vi "Savitsky Golay Weighted Filter (multiple).vi"(4 "Window Order":i32, 6 "Side Points Unit (points)":enum16{"Points", "Data"}(ring), 8 "error in (no error)":errorcluster, 9 "polynomial order (3)":i32=3, 10 "side points (6)":dbl=6.0, 11 "XY-data":cluster{"X-array":dbl[], "Y-array":dbl[]}[](array[cluster])) -> (0 "error out":errorcluster, 3 "XY-data out":cluster{"X-array":dbl[], "Y-array":dbl[]}[](array[cluster]) {"Y-array" format="%.2p"; "X-array" format="%.2p"})   [LabVIEW 2019, in "xy_utilities.lvlib"]
doc: "Filter <b>XY-data</b>'s Y-Array with a Savitsky-Golay FIR smoothing filter.\n\n<b>side points</b> specifies the number of data points to each side of the current data point to use for the least squares minimization. side points*2 + 1 is the length of the moving window, which must be greater than the polynomial order.\n\n<b>polynomial order</b> specifies the order of the polynomial. \n\nWire data to the data input to determine the polymorphic instance to use or manually select the instance."
uses:
  xy_utilities.lvlib
  Private/X Units.vi
  <vilib>/Analysis/3filter.llb/Savitzky-Golay Filter.vi
  <vilib>/Analysis/3filter.llb/Savitzky-Golay Filter (DBL).vi
  Private/X Array Range to Index.vi
  Private/Hann Windows.vi
  <vilib>/Utility/error.llb/Error Cluster From Error Code.vi
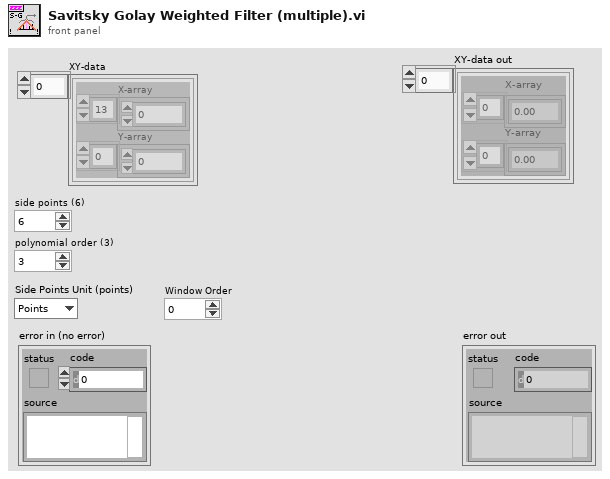
[diagram p1: front panel]
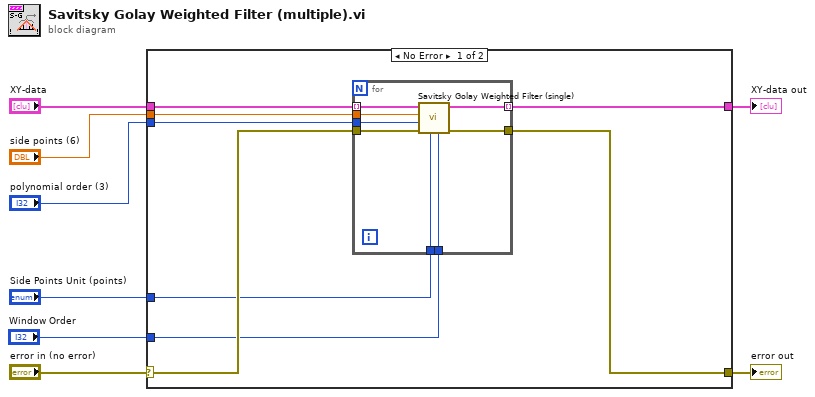
[diagram p0: block diagram]
diagram:
  n1 = case shown="No Error" "error in (no error)" {
    selector: "error in (no error)" -> [w13 w26]
    tunnel: [w12 w26] -> w7
    tunnel: "XY-data" -> [w16 w25]
    tunnel: [w15 w25] -> w5
    tunnel: "side points (6)" -> [w14 _]
    tunnel: "polynomial order (3)" -> [w11 _]
    tunnel: "Window Order" -> [w10 _]
    tunnel: "Side Points Unit (points)" -> [w9 _]
    frame No Error {
      n2 = for {
        tunnel: w16 -> [w24] mode=indexing
        tunnel: [w23] -> w15 mode=indexing
        tunnel: w14 -> [w22]
        tunnel: w13 -> [w21]
        tunnel: [w20] -> w12
        tunnel: w9 -> [w19]
        tunnel: w11 -> [w18]
        tunnel: w10 -> [w17]
        n3 = call "Savitsky Golay Weighted Filter (single).vi"("Window Order"=w17, "Side Points Unit (points)"=w19, "error in (no error)"=w21, "polynomial order (3)"=w18, "side points (6)"=w22, "XY-data"=w24) -> ("error out"=w20:errorcluster, "XY-data out"=w23:cluster{"X-array":dbl[], "Y-array":dbl[]})  [unwired: 4 in]
      }
    }
    frame Error {
    }
  }
  "error out" <- w7
  "XY-data out" <- w5
